vi "Update String Indicator From Ref.vi"(8 "Error In":errorcluster, 10 "String to Write":string, 11 "String Display Ref":refnum<vi>) -> (0 "Error Out":errorcluster)   [LabVIEW 2017]
doc: "This VI updates a string indicator given a reference to the indicator and the string value to place.\n\nParams:\nstring* String Display Ref -> string indicator to display message data\nstring String to Write -> message to update display to"
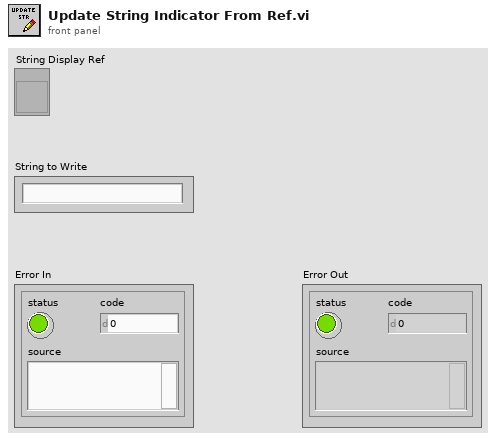
[diagram p1: front panel]
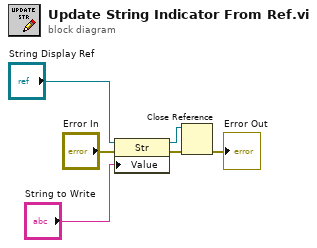
[diagram p0: block diagram]
diagram:
  n1 = property class="Str"(reference="String Display Ref", error in="Error In", "Value"="String to Write") -> (reference out=w2:refnum<vi>, error out=w3:errorcluster)
  n2 = Close Reference(reference=w2, error in (no error)=w3) -> (error out=→"Error Out":errorcluster)
